vi "SearchForLatestBinary.vi"(11 "Input string":string="i\u0000\u0000\u0000>\u0001\u0000\u0000AC_vxWorks_1.0.4.bin,AC_vxWorks_0.14.0.bin,AC_vxWorks_1.0.6.bin,AC_vxWorks_0.11.55.bin||PC_vxWorks_1.0.4.bin,PC_vxWorks_0.14.0.bin,PC_vxWorks_1.0.6.bin,PC_vxWorks_0.11.55.bin||SC_vxWorks_1.0.4_20khz.bin,SC_vxWorks.bin,SC_vxWorks_0.14.0.bin,SC_vxWorks_1.0.4.bin,SC_vxWorks_1.0.6_20khz.bin,SC_vxWorks_0.11.55_20khz.bin||") -> (3 "Output string":string)   [LabVIEW 2017]
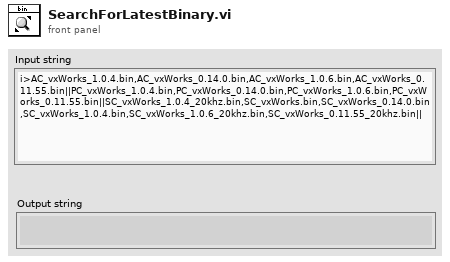
[diagram p1: front panel]
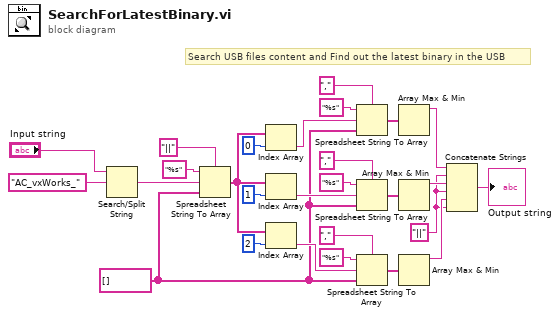
[diagram p0: block diagram]
diagram:
  w2 = "||"
  w6 = string[] [] ("array type (2D Dbl)")
  # "Search USB files content and Find out the latest binary in the USB"
  n1 = Search/Split String(string="Input string", search string/char (-)="AC_vxWorks_") -> (match + rest of string=w19:string)  [unwired: 1 in, 2 out]
  n2 = Spreadsheet String To Array(delimiter (Tab)="||", format string="%s", spreadsheet string=w19, array type (2D Dbl)=w6) -> (array=w7:string[])
  n3 = Index Array(array=w7, index=0) -> (element=w22:string)
  n4 = Index Array(array=w7, index=1) -> (element=w14:string)
  n5 = Index Array(array=w7, index=2) -> (element=w11:string)
  n6 = Spreadsheet String To Array(delimiter (Tab)=",", format string="%s", spreadsheet string=w22, array type (2D Dbl)=w6) -> (array=w18:string[])
  n7 = Spreadsheet String To Array(delimiter (Tab)=",", format string="%s", spreadsheet string=w14, array type (2D Dbl)=w6) -> (array=w17:string[])
  n8 = Spreadsheet String To Array(delimiter (Tab)=",", format string="%s", spreadsheet string=w11, array type (2D Dbl)=w6) -> (array=w8:string[])
  n9 = Array Max & Min(array=w18) -> (max value=w5:string)  [unwired: 3 out]
  n10 = Array Max & Min(array=w17) -> (max value=w4:string)  [unwired: 3 out]
  n11 = Array Max & Min(array=w8) -> (max value=w3:string)  [unwired: 3 out]
  n12 = Concatenate Strings(w5, w2, w4, w2, w3, w2) -> (→"Output string":string)
